vi "ma_Initial guess for tone estimation (FFT input).vi"(2 "spectral info":T1 {"window" items=["Rectangle"=0, "Hanning"=1, "Hamming"=2, "Blackman-Harris"=3, "Exact Blackman"=4, "Blackman"=5, "Flat Top"=6, "4 Term B-Harris "=7, "7 Term B-Harris"=8, "Low Sidelobe"=9, "Blackman Nuttall"=11, "Triangle"=30, "Bartlett-Hanning"=31, "Bohman"=32, "Parzen"=33, "Welch"=34, "Kaiser"=60, "Dolph-Chebyshev"=61, "Gaussian"=62]}, 3 "three fingers":T2={"f0"=0.0, "df"=1.0, "spectrum"=[]} {"spectrum" format="%.2f"; "df" format="%.2f"; "f0" format="%.2f"}) -> (0 "range":cluster{"f upper":dbl, "f lower":dbl} {"f lower" format="%.5f"; "f upper" format="%.5f"}, 1 "initial guess frequency":dbl format="%.9f")   [LabVIEW 2020, in "NI_MAPro.lvlib"]
uses:
  NI_MAPro.lvlib
  ma_sml_Spectrum Cluster (complex).ctl
  ma_sml_Spectral Info.ctl
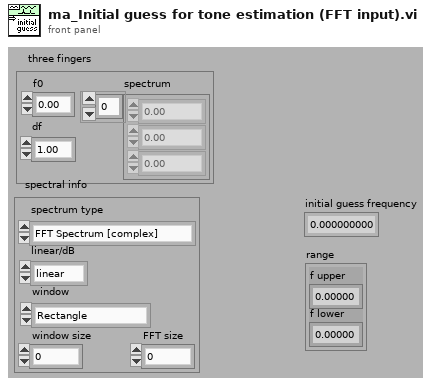
[diagram p1: front panel]
types:
  T1 = typedef "NI_MAPro.lvlib/ma_sml_Spectral Info.ctl" = cluster{"spectrum type":enum16{"FFT Spectrum [complex]", "Amplitude [Magnitude]", "Power [Magnitude^2]", "Cross Spectrum [complex]", "Frequency Response [Complex]"}, "linear/dB":enum16{"linear", "dB"}, "window":u16, "window size":i32, "FFT size":i32}
  T2 = typedef "NI_MAPro.lvlib/ma_sml_Spectrum Cluster (complex).ctl" = cluster{"f0":dbl, "df":dbl, "spectrum":cdb[]}
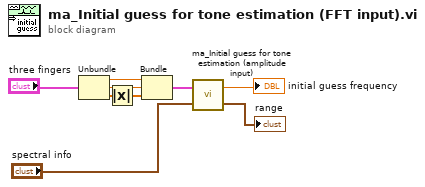
[diagram p0: block diagram]
diagram:
  n1 = Unbundle("three fingers") -> ("f0"=w7:dbl, "df"=w6:dbl, "spectrum"=w5:cdb[])
  n2 = Absolute Value(x=w5) -> (abs(x)=w3:dbl[])
  n3 = Bundle("f0"=w7, "df"=w6, w3) -> (w4:cluster{"f0":dbl, "df":dbl, dbl[]})  [unwired: 1 out]
  n4 = call "ma_Initial guess for tone estimation (amplitude input).vi"("spectral info"="spectral info", "three fingers"=w4) -> ("range"=→"range":cluster{"f upper":dbl, "f lower":dbl}, "initial guess frequecy"=→"initial guess frequency":dbl)
